vi "TelemetryServer_Shutdown.vi"(9 "error in (no error)":errorcluster) -> (6 "error out":errorcluster)   [LabVIEW 2009]
uses:
  TelemetryServer_Global.vi
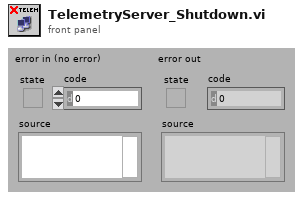
[diagram p1: front panel]
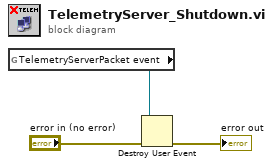
[diagram p0: block diagram]
diagram:
  n1 = global read "TelemetryServer_Global.vi" "TelemetryServerPacket event"() -> (w1:refnum<user-event>)
  n2 = Destroy User Event(user event=w1, error in="error in (no error)") -> (error out=→"error out":errorcluster)
